vi "ultrason.vi"() -> ()   [LabVIEW 2021]
uses:
  <vilib>/MakerHub/LINX/Public/Utilities/Open Serial.vi
  <vilib>/MakerHub/LINX/LMH-LINX.lvlib
  <vilib>/MakerHub/LINX/Public/Sensors/Distance/Ultrasonic/Ultrasonic.lvlib
panel:
  out "Distance (cm)":dbl(slide) scale=0.0..100.0
  in  "Serial Port":refnum<visa-resource-name>="N/A"
  out "Inches":dbl
  in  "stop":bool
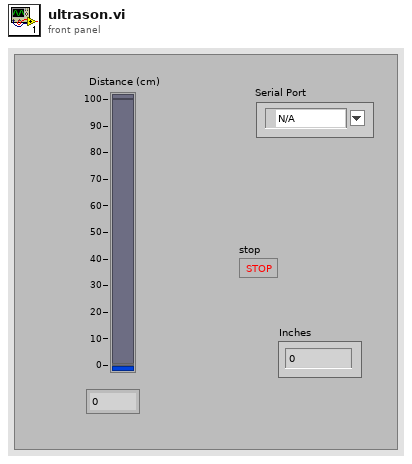
[diagram p1: front panel]
types:
  T1 = typedef "LMH-LINX.lvlib/LINX Ref.ctl" = cluster{"IO":T2, "Interface":T3, "LINX Device Config":T4}
  T2 = typedef "LMH-LINX.lvlib/Platform.ctl" = enum16{"Remote", "Local"}
  T3 = typedef "LMH-LINX.lvlib/Interface.ctl" = enum16{"Serial", "TCP"}
  T4 = typedef "LMH-LINX.lvlib/Device.lvlib/LINX Device Config.ctl" = cluster{"Interface":T3, "COM Port":refnum<visa-resource-name>, "TCP Configuration":T5, "Device Family":u8, "Device ID":u8, "Device Name":string, "TCP Ref":refnum<k5>, "Channels":T6}
  T5 = typedef "LMH-LINX.lvlib/Device.lvlib/TCP Config.ctl" = cluster{"IP Address":string, "Port":u16}
  T6 = typedef "LMH-LINX.lvlib/Channels.ctl" = cluster{"DI":u8[], "DO":u8[], "AI":u8[], "AO":u8[], "PWM":u8[], "QE":u8[], "UART":u8[], "I2C 2":u8[], "SPI":u8[], "CAN":u8[], "Servo":u8[], "AI Ref (V)":dbl, "AI Resolution (Bits)":u8, "AO Ref (V)":dbl, "AO Resolution (Bits)":u8}
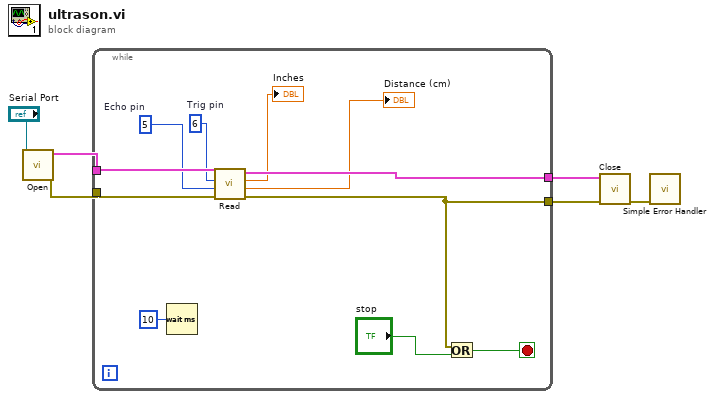
[diagram p0: block diagram]
diagram:
  n1 = call-poly <vilib>:"Open.vi"("Serial Port"="Serial Port") -> ("Error Out"=w5:errorcluster, "LINX Resource"=w6:T1)  [unwired: 8 in, 1 out]
  n2 = while {
    tunnel: w6 -> [w17]
    tunnel: w5 -> [w16]
    tunnel: [w12] -> w4
    tunnel: [w15] -> w3
    stop <- w14 stop-if-true
    w10 = u8 5  # Echo pin
    w11 = u8 6  # Trig pin
    n3 = Wait (ms)(milliseconds to wait=u32 10) -> ()  [unwired: 1 out]
    n4 = call <vilib>:"Read.vi"("Error In"=w16, "DO Channel"=w10, "DI Channel"=w11, "LINX Resource"=w17) -> ("Error Out"=w12:errorcluster, "Centimeters"=→"Distance (cm)":dbl, "Inches"=→"Inches":dbl, "LINX Resource"=w15:T1)  [unwired: 4 in]
    n5 = Or(x=w12, y="stop") -> (x .or. y?=w14:bool)
  }
  n6 = call <vilib>:"Close.vi"("Error In"=w4, "LINX Resource"=w3) -> ("Error Out"=w2:errorcluster)  [unwired: 9 in]
  n7 = call <vilib>:"Simple Error Handler.vi"("error in (no error)"=w2) -> ()  [unwired: 4 in, 5 out]
